vi "hpcnc reset if not idle.vi"(10 "error in (no error)":errorcluster, 11 "CNC COM in":refnum<visa-resource-name>) -> (0 "error out":errorcluster, 1 "CNC COM out":refnum<visa-resource-name>, 3 "Idle":bool)   [LabVIEW 2014]
uses:
  HPCNC.lvlib
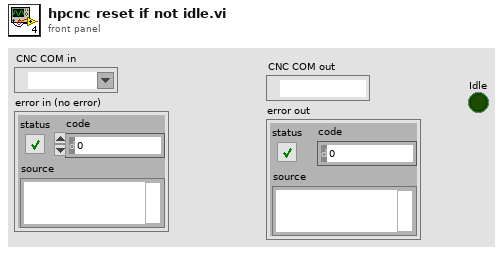
[diagram p1: front panel]
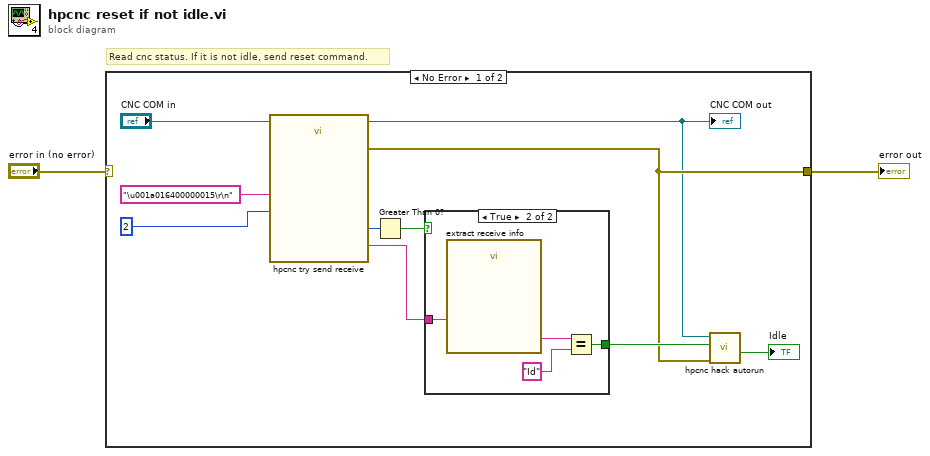
[diagram p0: block diagram]
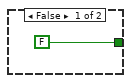
[diagram p2: hidden frame]
diagram:
  # "Read cnc status. If it is not idle, send reset command."
  n1 = case shown="No Error" "error in (no error)" {
    selector: "error in (no error)" -> [_ w18]
    tunnel: [w4 w18] -> w1
    frame No Error {
      n2 = call "hpcnc try send receive.vi"("Max try number"=2, "Send package"="\u001a016400000015\r\n" ("SendData"), "VISA Refnum in"="CNC COM in") -> ("error out"=w4:errorcluster, "Receive count"=w10:i32, "Receive package"=w11:string, "VISA Refnum out"=w3:refnum<visa-resource-name>)  [unwired: 5 in]
      "CNC COM out" <- w3
      n3 = Greater Than 0?(x=w10) -> (x > 0?=w9:bool)
      n4 = case shown="True" w9 {
        tunnel: w11 -> [_ w16]
        tunnel: [FALSE w15] -> w6
        frame False {
        }
        frame True {
          n5 = call "extract receive info.vi"("Receive data"=w16) -> ("STATUS"=w14:string)  [unwired: 11 in, 3 out]
          n6 = Equal?(x=w14, y="Id") -> (x = y?=w15:bool)
        }
      }
      n7 = call "hpcnc hack autorun.vi"("error in (no error)"=w4, "Idle"=w6, "VISA Refnum in"=w3) -> ("Reset"=→"Idle":bool)  [unwired: 7 in]
    }
    frame Error {
    }
  }
  "error out" <- w1
